vi "ComputeACPadPositions_Striptest.vi"(0 "Theta Calibration":dbl format="%#_8g", 1 "X cp":dbl format="%#_8g", 2 "Y cp":dbl format="%#_8g") -> ()   [LabVIEW 2019]
uses:
  <vilib>/Analysis/coordinate.llb/2D Cartesian Coordinate Rotation (Scalar).vi
  itk-strip-sensor-qc/LabVIEW 2019/QCtests/striptest/ProbePlan/ProbePlanParams.vi
  <vilib>/Analysis/NI_AALPro.lvlib
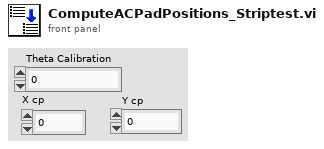
[diagram p1: front panel]
types:
  T1 = cluster{"Strip Number OUT":i32, "X0":i32, "Y0":i32, "X1":i32, "Y1":i32, "Xref":dbl, "Yref":dbl, "ProbePlan type":u32, "Inner pads offset":ext, "Outer pads offset":ext, "l_inner":ext, "l_outer":ext, "strip numbering":u16, "Device Orientation":ext, "Stagger offset":i32, "Yoffset":dbl, "Strip pitch":dbl, "Fiducail separation":dbl, "Radius":ext, "Relative strip angles":dbl, "Probeplan description":string, "ProbePlan array":cluster{"Region":string, "ProbePoints":cluster{"X":dbl, "Y":dbl, "Label":string, "CardViable?":bool}[]}[], "Test ProbePoints":cluster{"Regions Enabled":bool[], "From index":u32[], "To index":u32[]}}
  T2 = cluster{"Region":string, "ProbePoints":cluster{"X":dbl, "Y":dbl, "Label":string, "CardViable?":bool}[]}[]
  T3 = cluster{"X":dbl, "Y":dbl, "Label":string, "CardViable?":bool}[]
  T4 = cluster{"X":dbl, "Y":dbl, "Label":string, "CardViable?":bool}
  T5 = cluster{"Region":string, "ProbePoints":cluster{"X":dbl, "Y":dbl, "Label":string, "CardViable?":bool}[]}
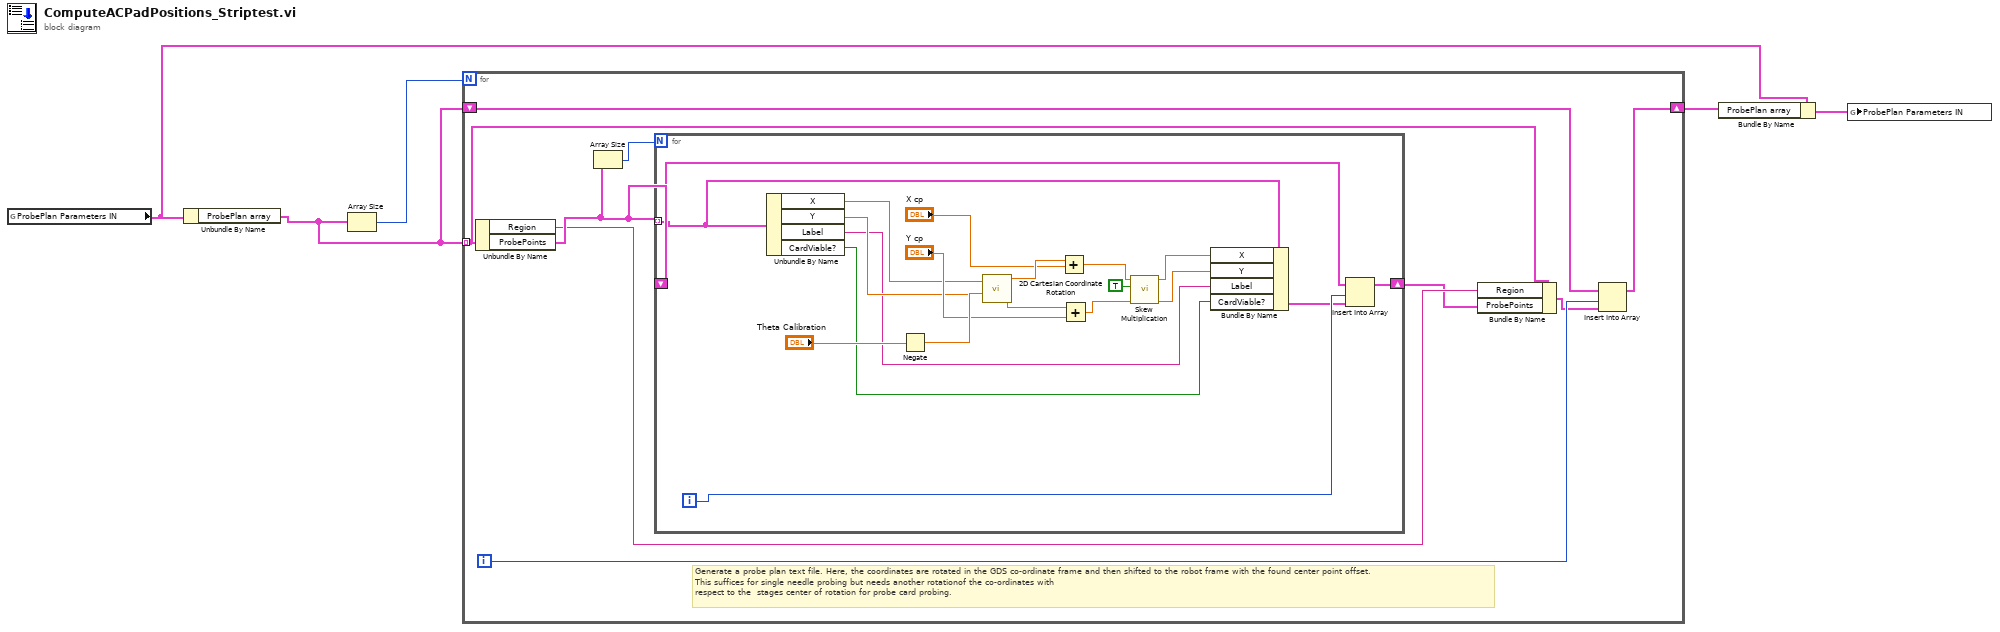
[diagram p0: block diagram]
diagram:
  n1 = global read "ProbePlanParams.vi" "ProbePlan Parameters IN"() -> (w3:T1)
  n2 = Unbundle By Name(w3) -> ("ProbePlan array"=w4:T2)
  n3 = Array Size(array=w4) -> (size(s)=w5:i32)
  n4 = for {
    N: w5 -> [_]
    tunnel: w4 -> [w9] mode=indexing
    shift-right: [w11] -> w2
    shift-left: w4 -> [w12]
    i -> [w10]
    # "Generate a probe plan text file. Here, the coordinates are rotated in the GDS co-ordinate frame and then shifted to the robot frame with the found center point offset. \nThis suffices for single needle probing but needs another rotationof the co-ordinates with\nrespect to the  stages center of rotation for probe card probing."
    n5 = Unbundle By Name(w9) -> ("Region"=w8:string, "ProbePoints"=w13:T3)
    n6 = Array Size(array=w13) -> (size(s)=w14:i32)
    n7 = for {
      N: w14 -> [_]
      tunnel: w13 -> [w19] mode=indexing
      shift-right: [w33] -> w7
      shift-left: w13 -> [w20]
      i -> [w34]
      n8 = Unbundle By Name(w19) -> ("X"=w23:dbl, "Y"=w22:dbl, "Label"=w16:string, "CardViable?"=w17:bool)
      n9 = Negate(x="Theta Calibration") -> (-x=w27:dbl)
      n10 = call-poly <vilib>:"2D Cartesian Coordinate Rotation.vi"("theta"=w27, "y"=w22, "x"=w23) -> ("y out"=w31:dbl, "x out"=w32:dbl)  [unwired: 6 in, 1 out]
      n11 = Add(x=w32, y="X cp") -> (x+y=w29:dbl)
      n12 = Add(x=w31, y="Y cp") -> (x+y=w28:dbl)
      n13 = call "Skew Multiplication.vi"("Y"=w28, "Boolean"=TRUE, "X"=w29) -> ("Y'"=w15:dbl, "X'"=w21:dbl)  [unwired: 7 in]
      n14 = Bundle By Name(cluster=w19, "X"=w21, "Y"=w15, "Label"=w16, "CardViable?"=w17) -> (w18:T4)
      n15 = Insert Into Array(array=w20, index=w34, new element=w18) -> (w33:T3)
    }
    n16 = Bundle By Name(cluster=w9, "Region"=w8, "ProbePoints"=w7) -> (w6:T5)
    n17 = Insert Into Array(array=w12, index=w10, new element=w6) -> (w11:T2)
  }
  n18 = Bundle By Name(cluster=w3, "ProbePlan array"=w2) -> (w1:T1)
  n19 = global write "ProbePlanParams.vi" "ProbePlan Parameters IN"(w1) -> ()
